vi "Motor_Open.vi"() -> ()   [LabVIEW 2016]
uses:
  <vilib>/Rock Robotics/SystemInterfaces/DIO/FPGA_DIOPWMChannel.ctl
  <vilib>/Rock Robotics/WPI/SafetyOutput/WPI_SafetyOutputConfigMenu.ctl
  <vilib>/Rock Robotics/WPI/MotorControl/WPI_MotorControlOpen Talon.vi
panel:
  in  "Right Motor 3 Inverted":bool=TRUE
  in  "Right Motor 2 Inverted":bool=TRUE
  in  "Right Motor 1 Inverted":bool=TRUE
  in  "Left Motor 3 Inverted":bool=TRUE
  in  "Left Motor 2 Inverted":bool=TRUE
  in  "Left Motor 1 Inverted":bool=TRUE
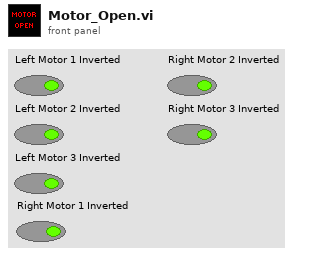
[diagram p1: front panel]
types:
  T1 = typedef "FPGA_DIOPWMChannel.ctl" = enum8{"PWM 0", "PWM 1", "PWM 2", "PWM 3", "PWM 4", "PWM 5", "PWM 6", "PWM 7", "PWM 8", "PWM 9", "PWM MXP 0", "PWM MXP 1", "PWM MXP 2", "PWM MXP 3", "PWM MXP 4", "PWM MXP 5", "PWM MXP 6", "PWM MXP 7", "PWM MXP 8", "PWM MXP 9", "Invalid"}
  T2 = typedef "WPI_SafetyOutputConfigMenu.ctl" = enum16{"Enable", "Disable"}
  T3 = typedef "WPI_RobotDriveDevRef.ctl" = cluster{"DevStatus":errorcluster, "Motors[]":T4[], "Square Inputs":bool, "Max Output":dbl}
  T4 = typedef "WPI_MotorControlDeviceRef.ctl" = cluster{"DeviceStatus":errorcluster, "Type":T5, "PWM":cluster{"PWM Channel":T1, "DeadBand":T6}, "CAN":cluster{"Device Number":u8, "SetOutput VI Ref":variant, "GetOutput VI Ref":variant, "Enable VI Ref":variant, "Disable VI Ref":variant, "Data":variant}, "Invert":bool}
  T5 = typedef "WPI_MotorControlType.ctl" = enum16{"PWM", "CAN"}
  T6 = typedef "WPI_PWMDeadband.ctl" = cluster{"Name":string, "maxPositivePwm":i32, "minPositivePwm":i32, "centerPwm":i32, "maxNegativePwm":i32, "minNegativePwm":i32, "angularRange":u16}
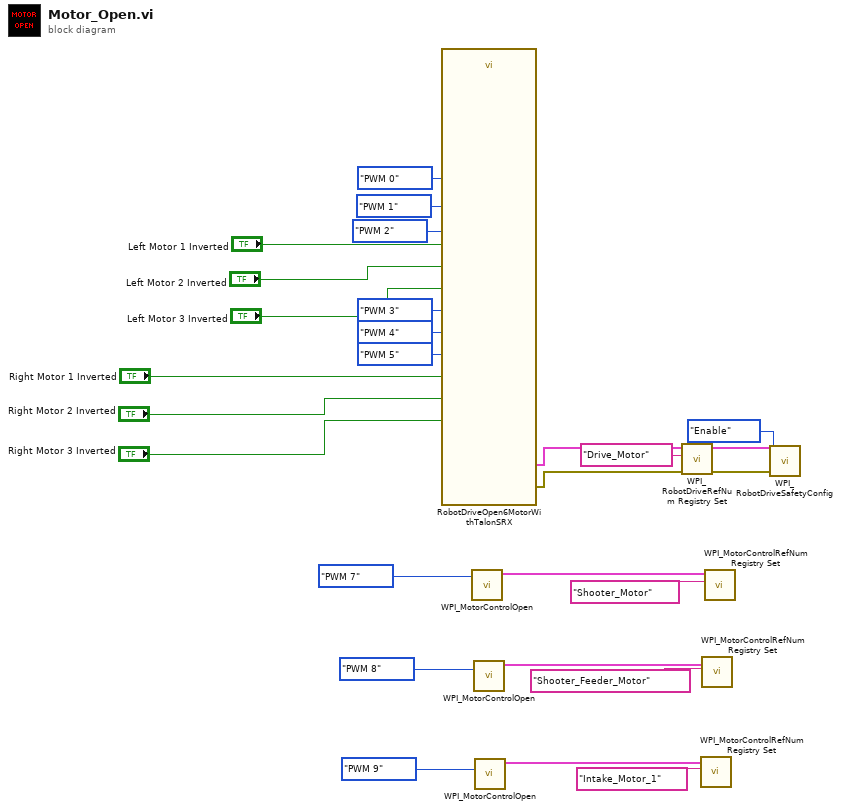
[diagram p0: block diagram]
diagram:
  n1 = call "RobotDriveOpen6MotorWithTalonSRX.vi"("Left Motor 1"=FPGA_DIOPWMChannel."PWM 0", "Left Motor 2"=FPGA_DIOPWMChannel."PWM 1", "Left Motor 3"=FPGA_DIOPWMChannel."PWM 2", "Right Motor 1"=FPGA_DIOPWMChannel."PWM 3", "Right Motor 2"=FPGA_DIOPWMChannel."PWM 4", "Right Motor 3"=FPGA_DIOPWMChannel."PWM 5", "Left Motor 1 Inverted"="Left Motor 1 Inverted", "Right Motor 1 Inverted"="Right Motor 1 Inverted", "Left Motor 2 Inverted"="Left Motor 2 Inverted", "Right Motor 2 Inverted"="Right Motor 2 Inverted", "Left Motor 3 Inverted"="Left Motor 3 Inverted", "Right Motor 3 Inverted"="Right Motor 3 Inverted") -> ("RobotDriveDevRef"=w11:T3, "error out"=w12:errorcluster)  [unwired: 14 in]
  n2 = call-poly <vilib>:"WPI_MotorControlOpen.vi"("PWM Channel"=FPGA_DIOPWMChannel."PWM 7") -> ("MotorControlDeviceRef"=w18:T4)  [unwired: 9 in, 1 out]
  n3 = call-poly <vilib>:"WPI_MotorControlOpen.vi"("PWM Channel"=FPGA_DIOPWMChannel."PWM 8") -> ("MotorControlDeviceRef"=w17:T4)  [unwired: 9 in, 1 out]
  n4 = call-poly <vilib>:"WPI_MotorControlOpen.vi"("PWM Channel"=FPGA_DIOPWMChannel."PWM 9") -> ("MotorControlDeviceRef"=w16:T4)  [unwired: 9 in, 1 out]
  n5 = call <vilib>:"WPI_RobotDriveRefNum Registry Set.vi"("error in (no error)"=w12, "refnum name"="Drive_Motor", "RobotDriveDevRef"=w11) -> ("error out"=w9:errorcluster, "RobotDriveDevRef"=w10:T3)  [unwired: 7 in]
  n6 = call <vilib>:"WPI_MotorControlRefNum Registry Set.vi"("refnum name"="Intake_Motor_1", "MotorControlDevRef"=w16) -> ()  [unwired: 8 in, 2 out]
  n7 = call <vilib>:"WPI_MotorControlRefNum Registry Set.vi"("refnum name"="Shooter_Feeder_Motor", "MotorControlDevRef"=w17) -> ()  [unwired: 8 in, 2 out]
  n8 = call <vilib>:"WPI_MotorControlRefNum Registry Set.vi"("refnum name"="Shooter_Motor", "MotorControlDevRef"=w18) -> ()  [unwired: 8 in, 2 out]
  n9 = call <vilib>:"WPI_RobotDriveSafetyConfig.vi"("error in (no error)"=w9, "mode"=WPI_SafetyOutputConfigMenu."Enable", "RobotDriveDevRef"=w10) -> ()  [unwired: 7 in, 2 out]
